vi "Assemble data for saving to buffer.vi"(10 "AOL_Globals":T1 {"Angle Ys (degrees)" format="%#.6g"; "Angle Xs (degrees)" format="%#.6g"; "Plane Mode" items=["XY Plane", "XZ Plane", "YZ Plane", "arbitraryplane"]; "Frame Size" items=["100X100"=100, "128X128"=128, "200X200"=200, "256X256"=256, "512X512"=512, "1024x1024"=1024, "2048x2048"=2048]; "Back Apperture (mA)" format="%#.6g"; "Pockels (V)" format="%#.6g"; "PMT 2" format="%#.6g"; "PMT 1" format="%#.6g"; "Angle (degrees)" format="%#.6g"; "POI Dwell time (us)" format="%#.6g"}, 11 "Stage XYZ Position":cluster{"X":sgl, "Y":sgl, "Z":sgl}) -> (3 "Imaging Parameters":T7)   [LabVIEW 2020]
uses:
  TypeDefs/Current Imaging Parameters.ctl
  Typedefs/Controls/AOL_Globals.ctl
  Typedefs/Imaging Protocols enum.ctl
  Typedefs/Frame Size.ctl
  Typedefs/AOL modes.ctl
  Typedefs/Plane Mode.ctl
  Typedefs/Functional Mode.ctl
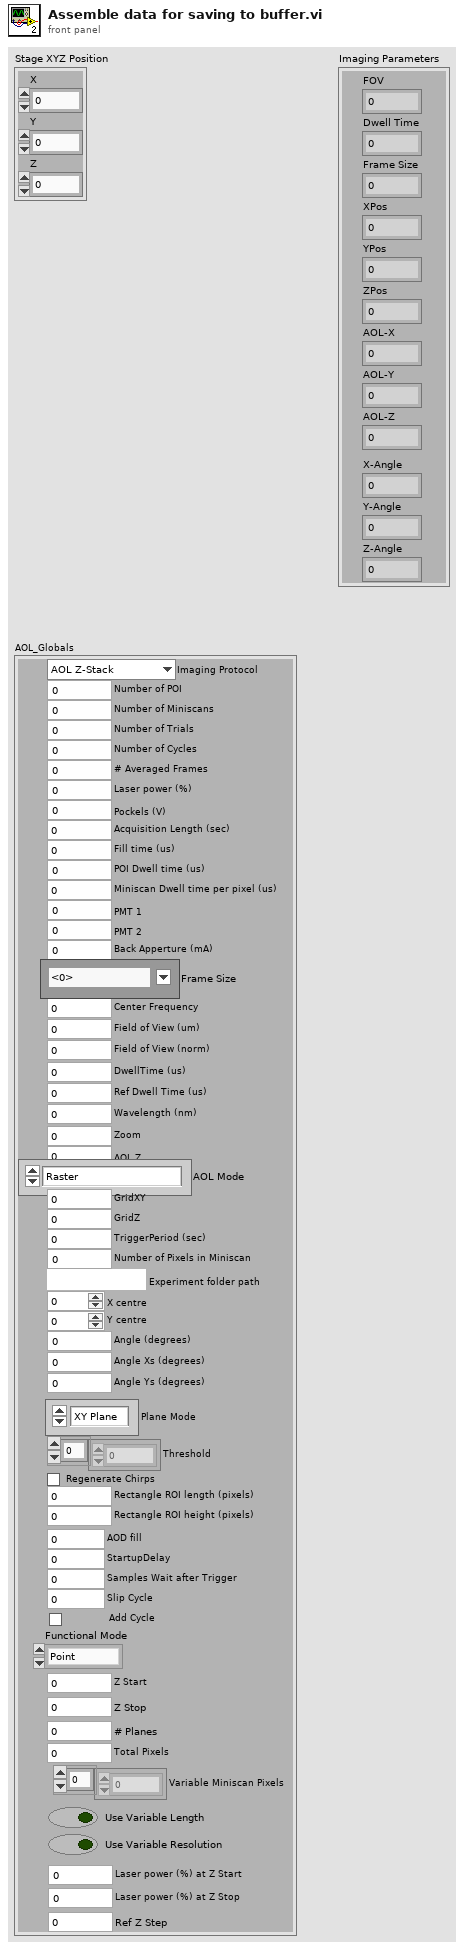
[diagram p1: front panel]
types:
  T1 = typedef "AOL_Globals.ctl" = cluster{"Imaging Protocol":T2, "Number of POI":u16, "Number of Miniscans":u16, "Number of Trials":u16, "Number of Cycles ":u64, "# Averaged Frames":u16, "Laser power (%)":u8, "Pockels (V)":dbl, "Acquisition Length (sec)":dbl, "Fill time (us)":dbl, "POI Dwell time (us)":dbl, "Miniscan Dwell time per pixel (us)":dbl, "PMT 1":dbl, "PMT 2":dbl, "Back Apperture (mA)":dbl, "Frame Size":T3, "Center Frequency":dbl, "Field of View (um)":dbl, "Field of View (norm)":dbl, "DwellTime (us)":dbl, "Ref Dwell Time (us)":dbl, "Wavelength (nm)":dbl, "Zoom":dbl, "AOL Z":dbl, "AOL Mode":T4, "GridXY":dbl, "GridZ":dbl, "TriggerPeriod (sec)":dbl, "Number of Pixels in Miniscan":u16, "Experiment folder path":path, "X centre":dbl, "Y centre":dbl, "Angle (degrees)":dbl, "Angle Xs (degrees)":dbl, "Angle Ys (degrees)":dbl, "Plane Mode":T5, "Threshold":u16[], "Regenerate Chirps":bool, "Rectangle ROI length (pixels)":u16, "Rectangle ROI height (pixels)":u16, "AOD fill":u16, "StartupDelay":i32, "Samples Wait after Trigger":u16, "Slip Cycle":u32, "Add Cycle":bool, "Functional Mode":T6, "Z Start":dbl, "Z Stop":dbl, "# Planes":i32, "Total Pixels":i32, "Variable Miniscan Pixels":u16[], "Use Variable Length":bool, "Use Variable Resolution":bool, "Laser power (%) at Z Start":u8, "Laser power (%) at Z Stop":u8, "Ref Z Step":i8}
  T2 = typedef "Imaging Protocols enum.ctl" = enum16{"AOL Z-Stack", "Motor Z Stack", "Parameter Sweep", "Functional Acquisition", "Single Plane Acquisition", "Volume Acquisition", "Live Imaging", "Live Plane Imaging", "Live Volume Imaging"}
  T3 = typedef "Frame Size.ctl" = u16
  T4 = typedef "AOL modes.ctl" = enum16{"Raster", "Structural", "Pointing", "Mini Scan", "Alignment"}
  T5 = typedef "Plane Mode.ctl" = u16
  T6 = typedef "Functional Mode.ctl" = enum16{"Point", "Line", "Patch", "Plane", "Volume"}
  T7 = typedef "Current Imaging Parameters.ctl" = cluster{"FOV":dbl, "Dwell Time":dbl, "Frame Size":dbl, "XPos":dbl, "YPos":dbl, "ZPos":dbl, "AOL-X":dbl, "AOL-Y":dbl, "AOL-Z":dbl, "X-Angle":dbl, "Y-Angle":dbl, "Z-Angle":dbl}
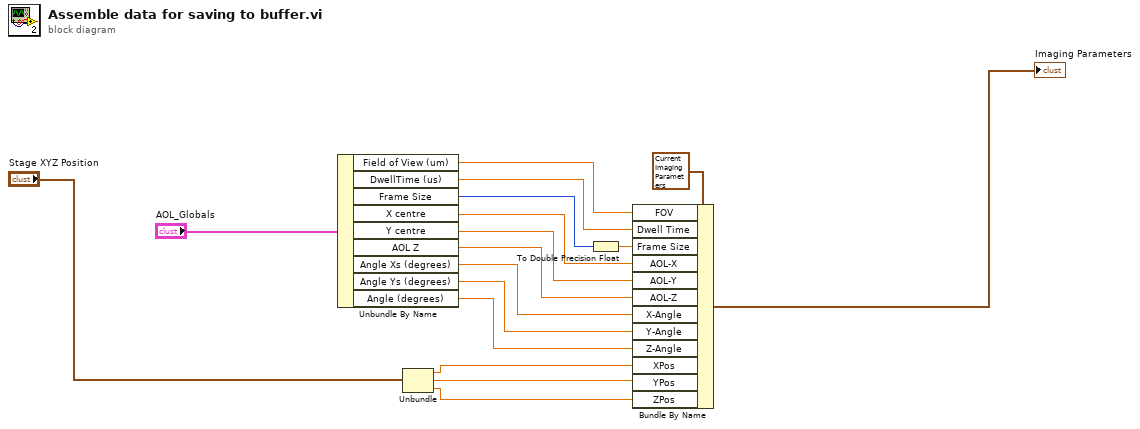
[diagram p0: block diagram]
diagram:
  n1 = Unbundle By Name("AOL_Globals") -> ("Field of View (um)"=w3:dbl, "DwellTime (us)"=w4:dbl, "Frame Size"=w5:T3, "X centre"=w7:dbl, "Y centre"=w8:dbl, "AOL Z"=w9:dbl, "Angle Xs (degrees)"=w10:dbl, "Angle Ys (degrees)"=w11:dbl, "Angle (degrees)"=w12:dbl)
  n2 = Unbundle("Stage XYZ Position") -> ("X"=w14:sgl, "Y"=w15:sgl, "Z"=w16:sgl)
  n3 = To Double Precision Float(number=w5) -> (double precision float=w6:dbl)
  n4 = Bundle By Name(cluster=T7 {"FOV"=0.0, "Dwell Time"=0.0, "Frame Size"=0.0, "XPos"=0.0, "YPos"=0.0, "ZPos"=0.0, "AOL-X"=0.0, "AOL-Y"=0.0, "AOL-Z"=0.0, "X-Angle"=0.0, "Y-Angle"=0.0, "Z-Angle"=0.0} ("Imaging Parameters"), "FOV"=w3, "Dwell Time"=w4, "Frame Size"=w6, "AOL-X"=w7, "AOL-Y"=w8, "AOL-Z"=w9, "X-Angle"=w10, "Y-Angle"=w11, "Z-Angle"=w12, "XPos"=w14, "YPos"=w15, "ZPos"=w16) -> (→"Imaging Parameters":T7)
